vi "总磷启动(子VI).vi"(11 "元素":T1(ring)) -> (0 "error out":T2={"status"=FALSE, "代码"=4, "source"=""} caption="错误输出" {"代码" items=["执行成功"=1, "执行失败，但不知道原因"=2, "命令请求条件错误"=3, "通讯超时"=4, "系统繁忙不能执行"=5, "系统故障"=6, "没有数据"=100]})   [LabVIEW 2016, in "MB SLAVE.lvlib"]
uses:
  MB SLAVE.lvlib
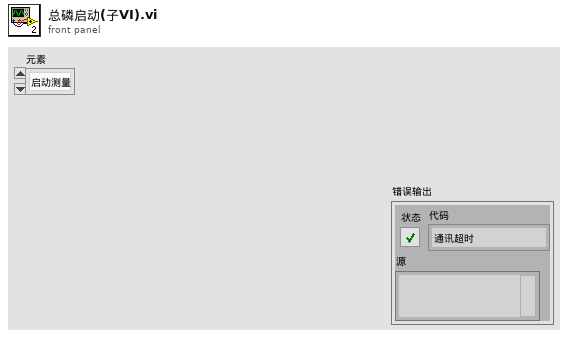
[diagram p1: front panel]
types:
  T1 = enum16{"启动测量", "标样核查", "零点核查", "跨度核查", "空白测试", "平行样测试", "加标回收", "空白校准", "标样校准", "初始化（清洗）", "停止测试", "仪器重启", "校时", "模式设置", "测量间隔设置"}
  T2 = cluster{"status":bool, "代码":u16, "source":string}
  T3 = enum16{"空闲", "水样测试", "标样核查", "零点核查", "跨度核查", "空白测试", "平行样测试", "加标回收", "空白校准", "标样校准", "初始化（清洗）"}
  T4 = typedef "总磷交互.ctl" = cluster{"状态告警区":cluster{"系统时间":timestamp, "工作状态":u16, "测量模式":enum16{"待机", "连续模式", "周期模式", "定点模式", "受控模式", "手动模式"}, "告警代码":u16, "故障代码":u16, "日志代码":u16, "软件版本":u16, "F0":sgl, "F1":sgl, "F2":sgl, "F3":sgl, "T":sgl, "H":sgl, "id":u16, "flowid":u16, "量程":u16, "总磷控温温度1":sgl, "营养盐控温温度2":sgl, "ADC":sgl}, "平台试剂余量百分比":sgl, "关键参数":cluster{"测量量程":dbl, "测量精度":dbl, "测量间隔":dbl, "消解温度":dbl, "消解时长":dbl, "空白校准时间":timestamp, "曲线截距":dbl, "曲线斜率":dbl, "测量检出限":dbl, "测量信号值":dbl, "线性相关系数":dbl, "二次多项式系数":dbl, "标样校准时间":timestamp, "稀释倍数":dbl, "三项式系数":dbl, "空白标定系数":dbl, "量程系数":dbl, "F0/ORPA":dbl, "F1/ORPB":dbl, "F2/ORPK":dbl, "F3":dbl, "F4":dbl, "F5":dbl, "F6":dbl, "F7":dbl, "X0/滴定数":dbl, "量程":dbl}, "关键参数改变":bool, "校准信息":cluster{"低标液1浓度":dbl, "低标液1信号值":dbl, "低标液1启用":u16, "低标液2浓度":dbl, "低标液2信号值":dbl, "低标液2启用":u16, "低标液3浓度":dbl, "低标液3信号值":dbl, "低标液3启用":u16, "低标液4浓度":dbl, "低标液4信号值":dbl, "低标液4启用":u16, "低标液5浓度":dbl, "低标液5信号值":dbl, "低标液5启用":u16, "高标液1浓度":dbl, "高标液1信号值":dbl, "高标液1启用":u16, "高标液2浓度":dbl, "高标液2信号值":dbl, "高标液2启用":u16, "高标液3浓度":dbl, "高标液3信号值":dbl, "高标液3启用":u16, "高标液4浓度":dbl, "高标液4信号值":dbl, "高标液4启用":u16, "高标液5浓度":dbl, "高标液5信号值":dbl, "高标液5启用":u16, "低斜率":dbl, "低截距":dbl, "低二次多项式系数":dbl, "低线性相关系数":dbl, "高斜率":dbl, "高截距":dbl, "高二次多项式系数":dbl, "高线性相关系数":dbl}, "校准信息改变":bool, "固件版本号":string}
  T5 = cluster{"站号":u16, "量程切换":enum32{"H", "L", "AUTO"}, "控制命令":enum16{"启动测量", "标样核查", "零点核查", "跨度核查", "空白测试", "平行样测试", "加标回收", "空白校准", "标样校准", "初始化（清洗）", "停止测试", "仪器重启", "校时", "模式设置", "测量间隔设置"}, "模式设置":enum16{"待机", "连续模式", "周期模式", "定点模式", "受控模式", "手动模式"}, "测量间隔":u16}
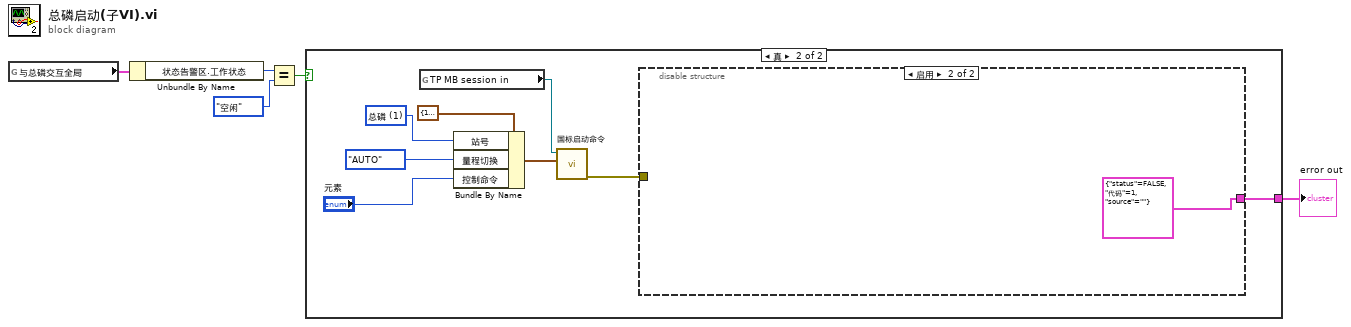
[diagram p0: block diagram]
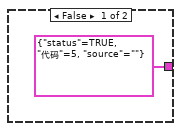
[diagram p2: hidden frame]
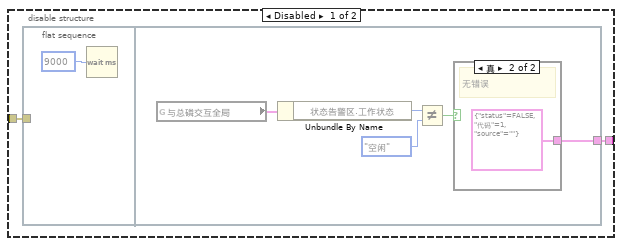
[diagram p3: hidden frame]
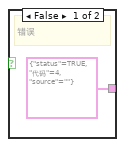
[diagram p4: hidden frame]
diagram:
  n1 = global read "modbus slave全局.vi" "与总磷交互全局"() -> (w2:T4)
  n2 = Unbundle By Name(w2) -> ("状态告警区.工作状态"=w1:u16)
  n3 = Equal?(x=w1, y=T3."空闲") -> (x = y?=w4:bool)
  n4 = case shown="真" w4 {
    tunnel: [T2 {"status"=TRUE, "代码"=5, "source"=""} ("error out") w14] -> w3
    frame False {
    }
    frame True {
      w11 = u16 1 items=["总磷"=1, "总氮"=2, "氨氮"=3, "CODMn"=21, "CODcr"=22, "氟化物"=50] ("站号")
      n5 = global read "modbus slave全局.vi" "TP MB session in"() -> (w9:refnum<class "MB_Master.lvclass">)
      n6 = Bundle By Name(cluster=T5 {"站号"=1, "量程切换"=enum."AUTO", "控制命令"=enum."启动测量", "模式设置"=enum."待机", "测量间隔"=0} ("参数"), "站号"=w11, "量程切换"=enum32{"H", "L", "AUTO"}."AUTO", "控制命令"="元素") -> (w13:T5)
      n7 = call "国标启动命令.vi"("参数"=w13, "MB session in"=w9) -> ("error out"=w7:errorcluster)  [unwired: 9 in]
      n8 = disable-structure shown="启用" {
        disable-tunnel: [w16 T2 {"status"=FALSE, "代码"=1, "source"=""} ("error out")] -> w14
        disable-tunnel: w7 -> [w15 _]
        frame Disabled {
          n9 = flat-sequence {
            tunnel: w15 -> [_]
            tunnel: [w22] -> w16
            frame #0 {
              n10 = Wait (ms)(milliseconds to wait=u32 9000 ("等待时间（毫秒）")) -> ()  [unwired: 1 out]
            }
            frame #1 {
              n11 = global read "modbus slave全局.vi" "与总磷交互全局"() -> (w19:T4)
              n12 = Unbundle By Name(w19) -> ("状态告警区.工作状态"=w18:u16)
              n13 = Not Equal?(x=w18, y=T3."空闲") -> (x != y?=w20:bool)
              n14 = case shown="真" w20 {
                tunnel: [T2 {"status"=TRUE, "代码"=4, "source"=""} ("error out") T2 {"status"=FALSE, "代码"=1, "source"=""} ("error out")] -> w22
                frame False {
                  # "错误"
                }
                frame True {
                  # "无错误"
                }
              }
            }
          }
        }
        frame Enabled {
        }
      }
    }
  }
  "error out" <- w3
